vi "Creator.vi"(9 "Is Priority":bool, 10 "Msg":refnum<class "Msg.lvclass">, 11 "Base Actor in":refnum<class "Base Actor.lvclass">) -> (3 "Base Actor out":refnum<class "Base Actor.lvclass">)   [LabVIEW 2020, in "jettl.lvlib" / "Actor.lvlib" / "Base Actor.lvclass"]
uses:
  Base Actor.lvclass
  Msg/Msg.lvclass
  Relation.ctl
  Actor.lvlib
  Error/Error.lvlib
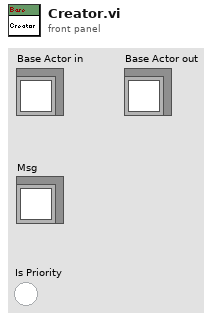
[diagram p1: front panel]
types:
  T1 = typedef "jettl.lvlib/Actor.lvlib/Attributes.ctl" = cluster{"Alias":string, "Address":refnum<user-event>, "Register":refnum<event-registration>, "Implemented Msgs":T2, "Path":path}
  T2 = typedef "jettl.lvlib/Actor.lvlib/Implemented Msgs.ctl" = set{refnum<class "Msg.lvclass">}
  T3 = typedef "jettl.lvlib/Actor.lvlib/Relation.ctl" = enum16{"Self", "Creator", "Created"}
  T4 = typedef "jettl.lvlib/Actor.lvlib/Error Info.ctl" = cluster{"Is Framework Error":bool, "Error":errorcluster}
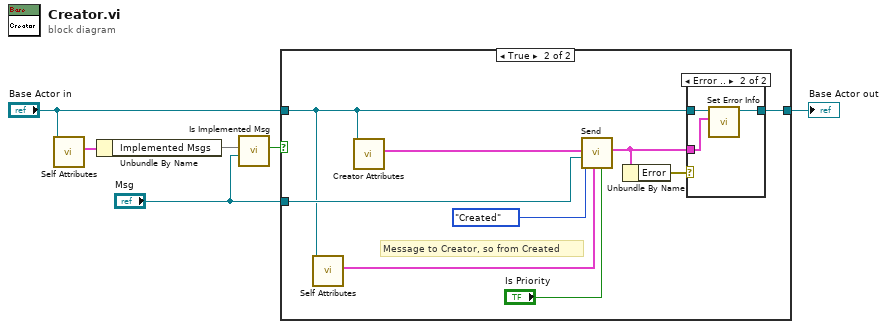
[diagram p0: block diagram]
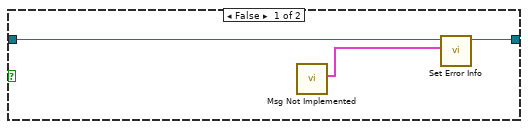
[diagram p2: hidden frame]
diagram:
  n1 = call-dynamic "Self Attributes.vi"("Base Actor in"="Base Actor in") -> ("Self Attributes"=w1:T1)  [unwired: 10 in]
  n2 = Unbundle By Name(w1) -> ("Implemented Msgs"=w4:T2)
  n3 = call "Is Implemented Msg.vi"("Msg"="Msg", "Implemented Msgs"=w4) -> ("Is Implemented Msg"=w5:bool)  [unwired: 9 in]
  n4 = case shown="True" w5 {
    tunnel: [w8 w10] -> w6
    tunnel: "Base Actor in" -> [w9 w11]
    tunnel: "Msg" -> [_ w15]
    frame False {
      n5 = call "Msg Not Implemented.vi"() -> ("Error Info"=w7:T4)  [unwired: 11 in]
      n6 = call "Set Error Info.vi"("Error Info"=w7, "Base Actor in"=w9) -> ("Base Actor out"=w8:refnum<class "Base Actor.lvclass">)  [unwired: 9 in]
    }
    frame True {
      # "Message to Creator, so from Created"
      n7 = call-dynamic "Self Attributes.vi"("Base Actor in"=w11) -> ("Self Attributes"=w16:T1)  [unwired: 10 in]
      n8 = call-dynamic "Creator Attributes.vi"("Base Actor in"=w11) -> ("Creator Attributes"=w18:T1)  [unwired: 10 in]
      n9 = call "Send.vi"("Is Priority"="Is Priority", "Self Attributes"=w16, "Relation"=Relation."Created", "Msg"=w15, "Attributes"=w18) -> ("Error Info"=w12:T4)  [unwired: 6 in]
      n10 = Unbundle By Name(w12) -> ("Error"=w13:errorcluster)
      n11 = case shown="Error .." w13 {
        tunnel: [w19 w21] -> w10
        tunnel: w11 -> [w19 w22]
        tunnel: w12 -> [_ w20]
        frame No Error {
        }
        frame Error {
          n12 = call "Set Error Info.vi"("Error Info"=w20, "Base Actor in"=w22) -> ("Base Actor out"=w21:refnum<class "Base Actor.lvclass">)  [unwired: 9 in]
        }
      }
    }
  }
  "Base Actor out" <- w6
